vi "Query Polarity.vi"(6 "channel":i32=1 min=1 max=4, 8 "error in (no error)":errorcluster, 11 "VISA resource name":refnum<visa-resource-name>) -> (0 "error out":errorcluster, 2 "polarity":T1 items=["Positive", "Negative"], 3 "VISA resource name out":refnum<visa-resource-name>)   [LabVIEW 2019, in "Pulse Rider PG-1000.lvlib"]
doc: "This command query the output polarity.\n\npolarity: the polarity: 'positive' or 'negative'\nchannel: the output channel int from 1 to 4"
uses:
  <instrlib>/Pulse Rider PG-1000/Pulse Rider PG-1000.lvlib
  <instrlib>/Pulse Rider PG-1000/Public/Configure/Pulse/Polarity.ctl
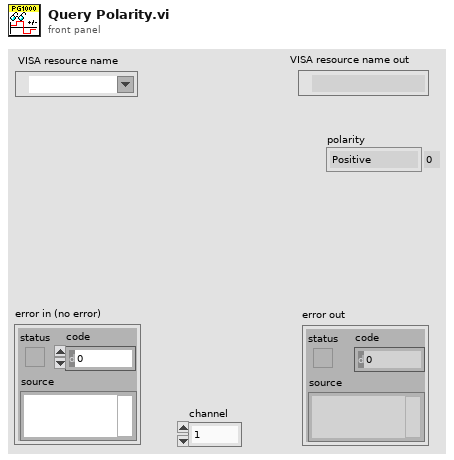
[diagram p1: front panel]
types:
  T1 = typedef "Pulse Rider PG-1000.lvlib/Polarity.ctl" = u16
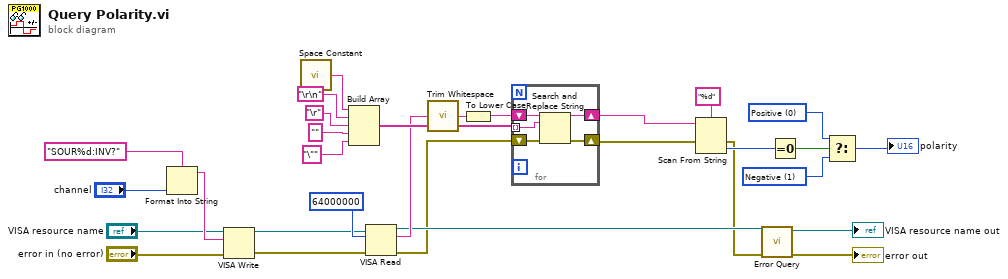
[diagram p0: block diagram]
diagram:
  w5 = T1 1 items=["Positive", "Negative"] ("Polarity (0: Positive)")
  w6 = T1 0 items=["Positive", "Negative"] ("Polarity (0: Positive)")
  n1 = Format Into String(format string="SOUR%d:INV?", "channel") -> (resulting string=w29:string)  [unwired: 2 in, 1 out]
  n2 = VISA Write(VISA resource name="VISA resource name", write buffer=w29, error in (no error)="error in (no error)") -> (VISA resource name out=w13:refnum<visa-resource-name>, error out=w11:errorcluster)  [unwired: 1 out]
  n3 = call <vilib>:"Space Constant.vi"() -> ("String"=w22:string)
  n4 = Build Array(w22, "\r\n", "\r", "", "\"") -> (w17:string[])
  n5 = VISA Read(VISA resource name=w13, byte count=u32 64000000, error in (no error)=w11) -> (VISA resource name out=w12:refnum<visa-resource-name>, read buffer=w15:string, error out=w3:errorcluster)  [unwired: 1 out]
  n6 = call <vilib>:"Trim Whitespace.vi"("string"=w15) -> ("trimmed string"=w16:string)  [unwired: 1 in]
  n7 = To Lower Case(string=w16) -> (all lower case string=w14:string)
  n8 = for {
    tunnel: w17 -> [w33] mode=indexing
    shift-right: [w35] -> w9
    shift-left: w14 -> [w34]
    shift-right: [w31] -> w2
    shift-left: w3 -> [w32]
    n9 = Search and Replace String(input string=w34, search string=w33, error in=w32) -> (result string=w35:string, error out=w31:errorcluster)  [unwired: 5 in, 2 out]
  }
  n10 = Scan From String(format string="%d", input string=w9, error in=w2) -> (error out=w1:errorcluster, output 1=w8:i32)  [unwired: 2 in, 2 out]
  n11 = call <instrlib>:"Error Query.vi"("error in (no error)"=w1, "VISA resource name"=w12) -> ("error out"=→"error out":errorcluster, "VISA resource name out"=→"VISA resource name out":refnum<visa-resource-name>)  [unwired: 6 in, 2 out]
  n12 = Equal To 0?(x=w8) -> (x = 0?=w7:bool)
  n13 = Select(t=w6, s=w7, f=w5) -> (s? t:f=→"polarity":T1)
